vi "Vbatt_SPI_Test.vi"() -> ()   [LabVIEW 2011]
uses:
  <vilib>/FPGAPlugInAG/sbRIO-9606/niLvFpga_Open_sbRIO-9606.vi
  <vilib>/Utility/error.llb/Error Cluster From Error Code.vi
  <vilib>/RVI Host/nirviSupport.llb/nirviErrorClusterFromErrorCode.vi
  <vilib>/rvi/errors/niLvFpgaAdjustHostInterfaceError.vi
  <vilib>/FPGAPlugInAG/sbRIO-9606/niLvFpga_Close_sbRIO-9606.vi
  <vilib>/rvi/interface/nirviOpenFPGA/nirviOpenFPGA.xnode
  SPI_TEST_REF.ctl
  FPGA Bitfiles/SailBot_FPGATarget3_VBattSenseSPITes_222C18A6.lvbitx
  1,3 A-Competition Platform/1,3 A Code/FPGA/VBattSense SPI Test.vi
  <vilib>/rvi/interface/nirviMethod/nirviMethod.xnode
  <vilib>/rvi/interface/nirviReadWriteControl/nirviReadWriteControl.xnode
  <vilib>/rvi/interface/nirviCloseFPGA/nirviCloseFPGA.xnode
  <vilib>/rvi/interface/nirviMethod/StockFPGA_InlinedMethodWaitForSingleIRQ.vi
  <vilib>/FPGAPlugInAG/sbRIO-9606/niLvFpga_WaitOnIrq_sbRIO-9606.vi
  <vilib>/FPGAPlugInAG/sbRIO-9606/niLvFpga_AcknowledgeIrq_sbRIO-9606.vi
  NiFpgaLv.dll
panel:
  in  "Wait Ticks":u32
  out "Battery Voltage":dbl(graph)
  in  "stop":bool
  out "error out":errorcluster
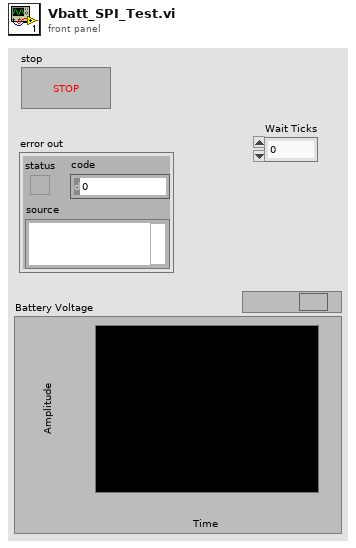
[diagram p1: front panel]
types:
  T1 = typedef "SPI_TEST_REF.ctl" = refnum<k20>
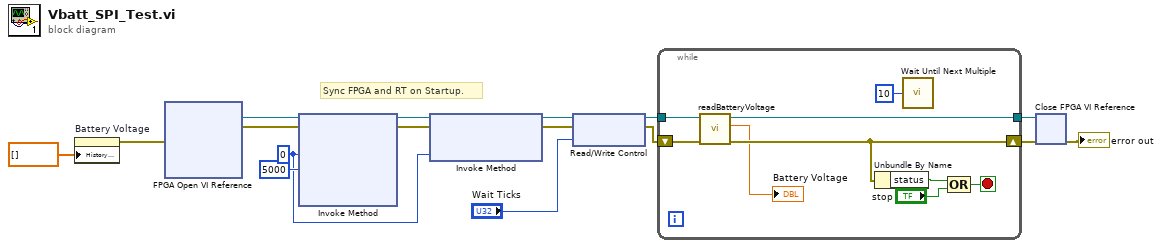
[diagram p0: block diagram]
diagram:
  w9 = 0 ("IRQ Number(s)")
  # "Sync FPGA and RT on Startup."
  n1 = property on="Battery Voltage" class="WFChart (strict)"("History Data"=dbl[] []) -> (error out=w2:errorcluster)  [unwired: 2 in, 1 out]
  n2 = xnode "FPGA Open VI Reference"("error in"=w2) -> ("FPGA VI Reference Out"=w14:T1, "error out"=w13:errorcluster)  [unwired: 1 in]
  n3 = xnode "Invoke Method"("FPGA VI Reference In"=w14, "error in"=w13, "IRQ Number(s)"=w9, "Timeout (ms)"=5000) -> ("FPGA VI Reference Out"=w12:T1, "error out"=w11:errorcluster)  [unwired: 2 out]
  n4 = xnode "Invoke Method"("FPGA VI Reference In"=w12, "error in"=w11, "IRQ Number(s)"=w9) -> ("FPGA VI Reference Out"=w7:T1, "error out"=w6:errorcluster)
  n5 = xnode "Read/Write Control"("FPGA VI Reference In"=w7, "error in"=w6, "Wait Ticks"="Wait Ticks") -> ("FPGA VI Reference Out"=w5:T1, "error out"=w4:errorcluster)
  n6 = while {
    tunnel: w5 -> [w22]
    tunnel: [w20] -> w16
    shift-right: [w19] -> w8
    shift-left: w4 -> [w21]
    stop <- w24 stop-if-true
    n7 = call "readBatteryVoltage.vi"("error in (no error)"=w21, "Refnum in"=w22) -> ("error out"=w19:errorcluster, "Battery Voltage (V)"=→"Battery Voltage":dbl, "Refnum out"=w20:T1)  [unwired: 7 in]
    n8 = Unbundle By Name(w19) -> ("status"=w18:bool)
    n9 = call "Wait Until Next Multiple"("Count(mSec)"=u32 10) -> ()  [unwired: 1 out]
    n10 = Compound Arithmetic op=OR(w18, "stop") -> (w24:bool)
  }
  n11 = xnode "Close FPGA VI Reference"("FPGA VI Reference In"=w16, "error in"=w8) -> ("error out"=→"error out":errorcluster)
